vi "WPI_DashboardAdd File Length.vi"(10 "String in":string, 11 "appended path":path) -> (2 "Valid":bool, 3 "String out":string)   [LabVIEW 2017]
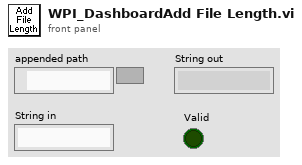
[diagram p1: front panel]
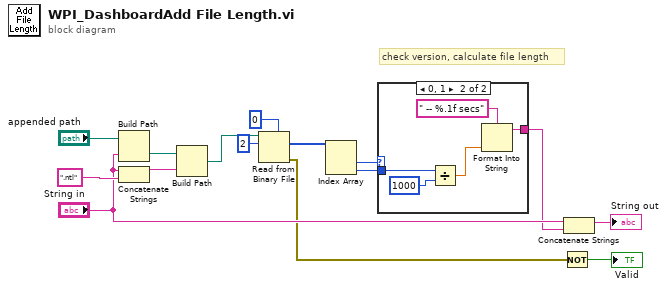
[diagram p0: block diagram]
diagram:
  # "check version, calculate file length"
  n1 = Build Path(base path="appended path", name or relative path="String in") -> (appended path=w6:path)
  n2 = Concatenate Strings("String in", ".ntl" ("string")) -> (w7:string)
  n3 = Build Path(base path=w6, name or relative path=w7) -> (appended path=w5:path)
  n4 = Read from Binary File(5:0, 10:2 ("count (1)"), 11:w5) -> (0:w4:errorcluster, 2:w11:i32[])  [unwired: 3 in, 2 out]
  n5 = Index Array(array=w11) -> (element #1=w2:i32, element #2=w10:i32)  [unwired: 2 in]
  n6 = case shown="0, 1" w2 {
    tunnel: w10 -> [_ w19]
    tunnel: [_ w16] -> w1
    frame Default {
    }
    frame 0, 1 {
      n7 = Divide(x=w19, y=1000) -> (x/y=w18:dbl)
      n8 = Format Into String(format string=" -- %.1f secs", w18) -> (resulting string=w16:string)  [unwired: 2 in, 1 out]
    }
  }
  n9 = Not(x=w4) -> (.not. x?=→"Valid":bool)
  n10 = Concatenate Strings("String in", w1) -> (→"String out":string)
